vi "AddStepRun.vi"(5 "EndDate (Now)":timestamp, 6 "StepExecutionStatus (NOT_COMPLETED)":T1=enum."NOT_COMPLETED", 7 "StartDate (Now)":timestamp, 8 "error in":errorcluster, 10 "StepName":string, 11 "SequenceRun in":refnum<class "SequenceRun.lvclass">) -> (0 "error out":errorcluster, 2 "StepRun":refnum<class "StepRun.lvclass">, 3 "SequenceRun out":refnum<class "SequenceRun.lvclass">)   [LabVIEW 2021, in "ProligentXMLGenerator.lvlib" / "SequenceRun.lvclass"]
doc: "Add a StepRun.\n\nA step run is a time-bound logical container for a set of measures.\nA step run is uniquely identified by its StepRunId."
uses:
  SequenceRun.lvclass
  SequenceRun.lvclass/SequenceRun.ctl
  StepRun/StepRun/StepRun.lvclass
  Base/ExecutionStatus/Value.ctl
  Base/ExecutionStatus/ExecutionStatus.lvclass
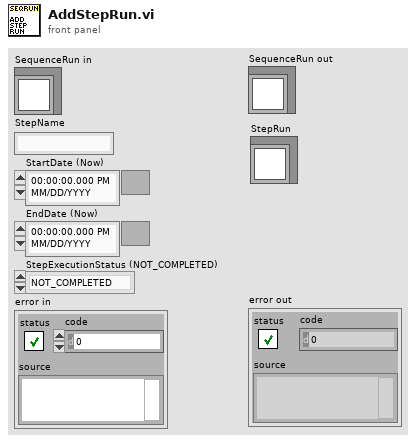
[diagram p1: front panel]
types:
  T1 = typedef "ProligentXMLGenerator.lvlib/ExecutionStatus.lvclass/Value.ctl" = enum16{"PASS", "FAIL", "NOT_COMPLETED", "ABORTED"}
  T2 = typedef "ProligentXMLGenerator.lvlib/SequenceRun.lvclass/Data.ctl" = cluster{"Name":string, "StepRuns":refnum<class "StepRun.lvclass">[], "Characteristics":refnum<class "Characteristic.lvclass">[], "Documents":refnum<class "Document.lvclass">[], "FailureReferences":refnum<class "FailureReference.lvclass">[], "CustomData":refnum<class "CustomData.lvclass">, "StartDate":refnum<class "DateTime.lvclass">, "EndDate":refnum<class "DateTime.lvclass">, "SequenceExecutionStatus":refnum<class "ExecutionStatus.lvclass">, "SequenceRunId":refnum<class "Guid.lvclass">, "SequenceFullName":refnum<class "SequenceFullName.lvclass">, "SequenceVersion":refnum<class "NonEmptyString_64.lvclass">, "StationFullName":refnum<class "FullName.lvclass">, "User":refnum<class "NonEmptyString_255.lvclass">, "TimeZoneInfoId":string}
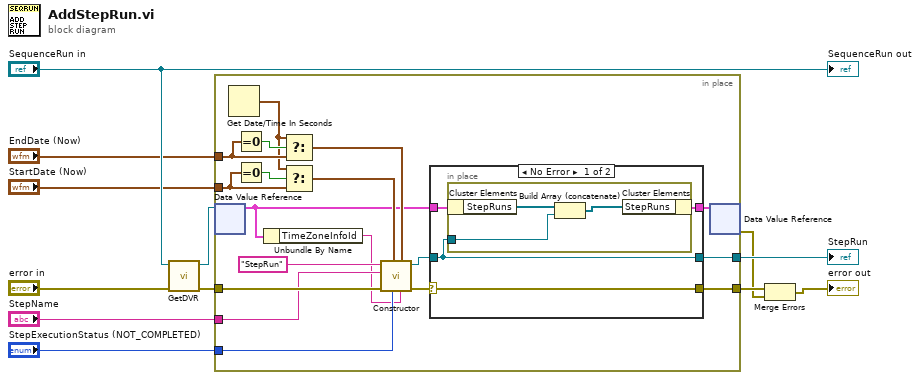
[diagram p0: block diagram]
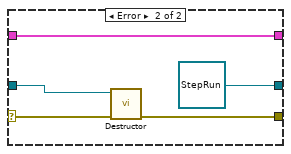
[diagram p2: hidden frame]
diagram:
  n1 = call "GetDVR.vi"("error in"="error in", "SequenceRun"="SequenceRun in") -> ("error out"=w4:errorcluster, "DVRReference"=w3:refnum<data-value>)  [unwired: 8 in]
  n2 = in-place "In Place Element Structure" {
    in-place-border: "StepName" -> [w23]
    in-place-border: [w29] -> w5
    in-place-border: w4 -> [w28]
    in-place-border: [w26] -> w8
    in-place-border: "StartDate (Now)" -> [w20]
    in-place-border: "StepExecutionStatus (NOT_COMPLETED)" -> [w22]
    in-place-border: "EndDate (Now)" -> [w16]
    n3 = in-place-dvr #1(w3) -> (w14:T2)  [unwired: 1 out]
    n4 = Get Date/Time In Seconds() -> (seconds since 1Jan1904=w15:timestamp)
    n5 = Equal To 0?(x=w16) -> (x = 0?=w19:bool)
    n6 = Equal To 0?(x=w20) -> (x = 0?=w21:bool)
    n7 = Unbundle By Name(w14) -> ("TimeZoneInfoId"=w13:string)
    n8 = Select(t=w15, s=w19, f=w16) -> (s? t:f=w18:timestamp)
    n9 = Select(t=w15, s=w21, f=w20) -> (s? t:f=w17:timestamp)
    n10 = call "Constructor.vi"("TimeZoneInfoId"=w13, "EndDate"=w18, "StepExecutionStatus"=w22, "StartDate"=w17, "error in"=w28, "StepName"=w23, "Name"="StepRun") -> ("error out"=w30:errorcluster, "StepRun out"=w25:refnum<class "StepRun.lvclass">)  [unwired: 3 in]
    n11 = case shown="No Error" w30 {
      selector: w30 -> [w34 w41]
      tunnel: [w31 w42] -> w27
      tunnel: [w34 w40] -> w29
      tunnel: w25 -> [w33 w39]
      tunnel: w14 -> [w32 w42]
      tunnel: [w33 refnum<class "StepRun.lvclass"> refnum ("ProligentResultProcessor:StepRun")] -> w26
      frame No Error {
        n12 = in-place "In Place Element Structure" {
          in-place-border: w33 -> [w37]
          n13 = in-place-cluster #2(w32) -> ("StepRuns"=w36:refnum<class "StepRun.lvclass">[])
          n14 = Build Array (concatenate)(w36, w37) -> (w35:refnum<class "StepRun.lvclass">[])
          n15 = in-place-cluster #2("StepRuns"=w35) -> (w31:T2)
        }
      }
      frame Error {
        n16 = call "Destructor.vi"("error in"=w41, "StepRun"=w39) -> ("error out"=w40:errorcluster)  [unwired: 9 in]
      }
    }
    n17 = in-place-dvr #1(w27) -> (w2:errorcluster)  [unwired: 1 out]
  }
  "StepRun" <- w8
  n18 = Merge Errors(w5, w2) -> (→"error out":errorcluster)
  "SequenceRun out" <- "SequenceRun in"
